vi "initialize.vi"(8 "error in (no error)":errorcluster, 11 "ReadyState in":refnum<class "ReadyState.lvclass">) -> (0 "error out":errorcluster, 3 "ReadyState out":refnum<class "ReadyState.lvclass">)   [LabVIEW 2016, in "ReadyState.lvclass"]
uses:
  ReadyState.lvclass
  State.lvclass
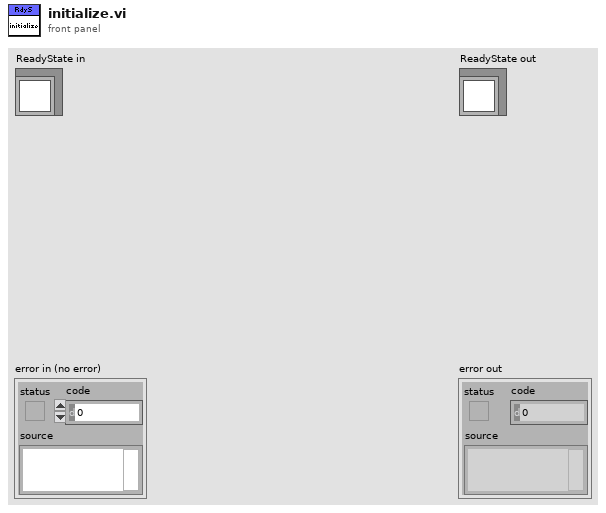
[diagram p1: front panel]
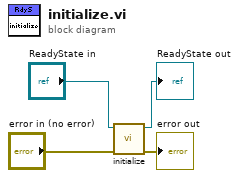
[diagram p0: block diagram]
diagram:
  n1 = call-parent "initialize.vi"("error in (no error)"="error in (no error)", "State in"="ReadyState in") -> ("error out"=→"error out":errorcluster, "State out"=→"ReadyState out":refnum<class "ReadyState.lvclass">)  [unwired: 8 in]
